vi "COM Interface.vi"() -> ()   [LabVIEW 2016]
uses:
  <vilib>/Instr/_visa.llb/VISA Configure Serial Port (Instr).vi
panel:
  out "Status":bool
  in  "Exit":bool
  in  "Connect":bool
  in  "COM port:":refnum<visa-resource-name>
  out "Answer":string
  in  "Send":bool
  in  "Command":string
  # "Update parameter string is:\nU=UPDATE\nnn = PARAM NUMBER\nL = LAYER\npp = VALUE\n\n- there is a space among them"
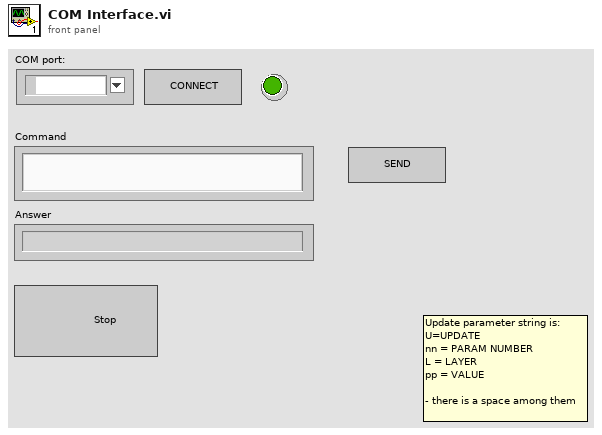
[diagram p1: front panel]
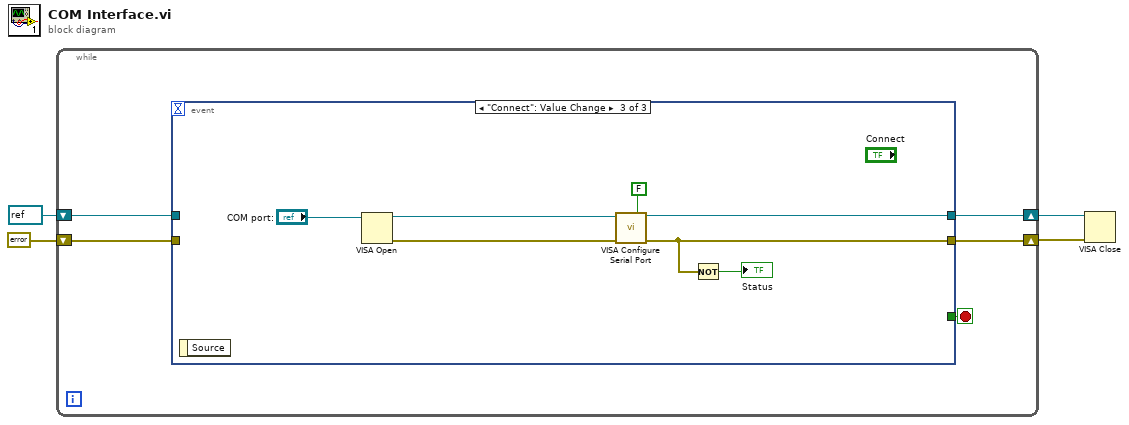
[diagram p0: block diagram]
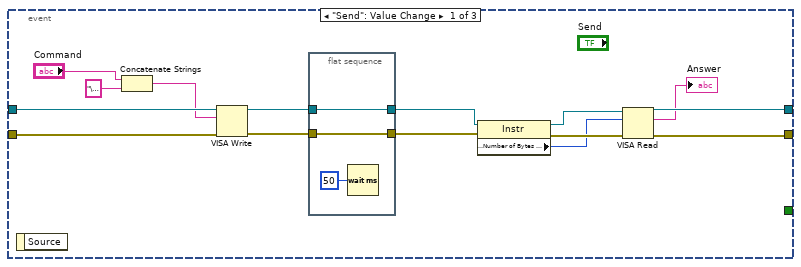
[diagram p2: hidden frame]
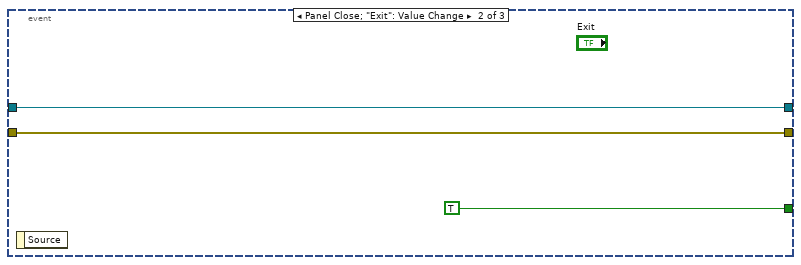
[diagram p3: hidden frame]
diagram:
  n1 = while {
    shift-right: [w7] -> w4
    shift-left: errorcluster {"status"=FALSE, "code"=0, "source"=""} ("error out") -> [w8]
    shift-right: [w6] -> w3
    shift-left: refnum<visa-resource-name> refnum ("VISA resource name out") -> [w5]
    stop <- w9 stop-if-true
    n2 = event shown="[2] \"Connect\": Value Change" {
      selector: _ -> [_ _ _]
      dyn-events: _ -> [_ _ _]
      timeout: _ -> [_ _ _]
      tunnel: [_ TRUE _] -> w9
      tunnel: w8 -> [w24 w29 _]
      tunnel: [w22 w28 w34] -> w6
      tunnel: [w21 w29 w33] -> w7
      tunnel: w5 -> [w23 w28 _]
      event "Send": Value Change {
        n3 = event-data() -> ()  [unwired: 1 in, 1 out]
        n4 = Concatenate Strings("Command", "\u0006") -> (w15:string)
        n5 = VISA Write(VISA resource name=w23, write buffer=w15, error in (no error)=w24) -> (VISA resource name out=w11:refnum<visa-resource-name>, error out=w13:errorcluster)  [unwired: 1 out]
        n6 = flat-sequence {
          tunnel: w13 -> [w26]
          tunnel: [w26] -> w12
          tunnel: [w25] -> w10
          tunnel: w11 -> [w25]
          frame #0 {
            n7 = Wait (ms)(milliseconds to wait=u32 50) -> ()  [unwired: 1 out]
          }
        }
        n8 = property class="Instr"(reference=w10, error in=w12) -> (reference out=w19:refnum<visa-resource-name>, error out=w20:errorcluster, "Serial Settings:Number of Bytes at Serial Port"=w18:u32)
        n9 = VISA Read(VISA resource name=w19, byte count=w18, error in (no error)=w20) -> (VISA resource name out=w22:refnum<visa-resource-name>, read buffer=→"Answer":string, error out=w21:errorcluster)  [unwired: 1 out]
      }
      event Panel Close; "Exit": Value Change {
        n10 = event-data() -> ()  [unwired: 1 in, 1 out]
      }
      event "Connect": Value Change {
        n11 = event-data() -> ()  [unwired: 1 in, 1 out]
        n12 = VISA Open(VISA resource name="COM port:") -> (VISA resource name=w36:refnum<visa-resource-name>, error out=w35:errorcluster)  [unwired: 4 in]
        n13 = call-poly "VISA Configure Serial Port"("VISA resource name"=w36, "Enable Termination\nChar (T)"=FALSE ("Enable Termination\nChar (T)"), "error in (no error)"=w35) -> ("VISA resource name out"=w34:refnum<visa-resource-name>, "error out"=w33:errorcluster)  [unwired: 11 in]
        n14 = Not(x=w33) -> (.not. x?=→"Status":bool)
      }
    }
  }
  n15 = VISA Close(VISA resource name=w3, error in (no error)=w4) -> ()  [unwired: 1 out]
